vi "region_of_interest.vi"() -> ()   [LabVIEW 2011]
uses:
  <vilib>/vision/Image Controls.llb/IMAQ Image.ctl
  <vilib>/vision/NI_Vision_Development_Module.lvlib
panel:
  out "Image Out 2":T1(plugin-control)
  out "Image Dst Out":T1
  out "Image Out":T1(plugin-control)
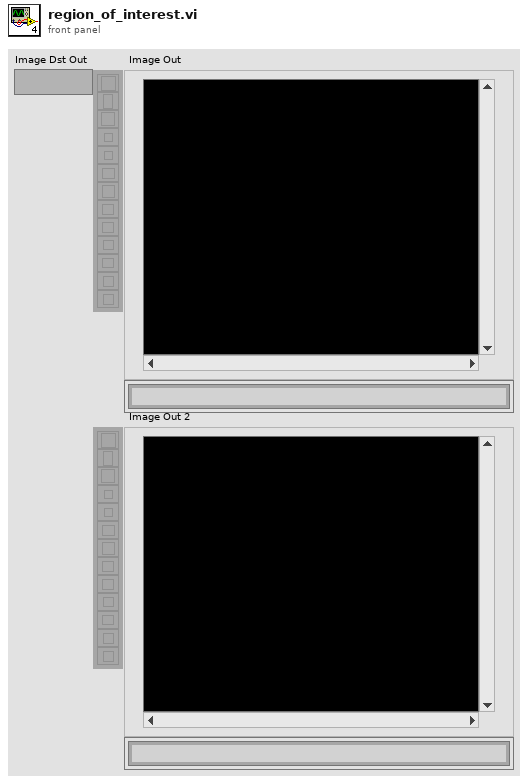
[diagram p1: front panel]
types:
  T1 = typedef "IMAQ Image.ctl" = refnum<image>
  T2 = typedef "IMAQ Rectangle" = cluster{"Left":i32, "Top":i32, "Right":i32, "Bottom":i32, "Rotation":dbl}
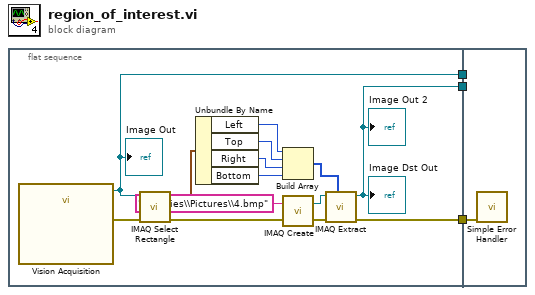
[diagram p0: block diagram]
diagram:
  n1 = flat-sequence {
    tunnel: [w7] -> w3
    tunnel: [w6] -> w2
    tunnel: [w5] -> w1
    tunnel: w3 -> [_]
    tunnel: w2 -> [w18]
    tunnel: w1 -> [_]
    frame #0 {
      n2 = call "Vision Acquisition"() -> ("Image Out"=w7:T1, "error out"=w17:errorcluster)  [unwired: 26 in]
      "Image Out" <- w7
      n3 = call "IMAQ Select Rectangle"("error in (no error)"=w17, "Image In"=w7) -> ("error out"=w11:errorcluster, "Rectangle"=w16:T2)  [unwired: 6 in, 2 out]
      n4 = Unbundle By Name(w16) -> ("Left"=w15:i32, "Top"=w14:i32, "Right"=w13:i32, "Bottom"=w12:i32)
      n5 = Build Array(w15, w14, w13, w12) -> (w10:i32[])
      n6 = call "IMAQ Create"("Image Name"="Libraries\\Pictures\\4.bmp", "error in (no error)"=w11) -> ("New Image"=w9:T1, "error out"=w8:errorcluster)  [unwired: 3 in]
      n7 = call "IMAQ Extract"("Optional Rectangle"=w10, "error in (no error)"=w8, "Image Src"=w9) -> ("error out"=w6:errorcluster, "Image Dst Out"=w5:T1)  [unwired: 7 in]
      "Image Dst Out" <- w5
      "Image Out 2" <- w5
    }
    frame #1 {
      n8 = call <vilib>:"Simple Error Handler.vi"("error in (no error)"=w18) -> ()  [unwired: 4 in, 5 out]
    }
  }
